vi "Do Action.vi"(8 "error in (no error)":errorcluster, 11 "Stand in":refnum<class "Stand.lvclass">) -> (0 "error out":errorcluster, 3 "Stand out":refnum<class "Stand.lvclass">)   [LabVIEW 2019, in "Stand.lvclass"]
uses:
  Stand.lvclass
  C:/Users/ANENKOV_V1/Desktop/src/Device_class/Device.lvclass
  Stand.lvclass/Stand.ctl
  TypeDef/Action.ctl
  FPGA/TypeDef/DO index.ctl
  Device_class/Device.lvclass/Device.ctl
  TypeDef/Active Motor.ctl
  TypeDef/Motor N.ctl
  AO_class/AO.lvclass/AO.ctl
  AI_class/AI.lvclass/AI.ctl
  AnalogComparator_class/AnalogComparator.lvclass/AnalogComparator.ctl
  OscillationClass/OscillationDetector.lvclass/OscillationDetector.ctl
  Valve_2DO_2DI_class/CMD.ctl
  NeedleValve_class/Cmd.ctl
  FPGA/TypeDef/AI index.ctl
  PM_Group_class/PM_Group.lvclass/PM_Group.ctl
  NeedleValve_class/NeedleValve.lvclass/NeedleValve.ctl
  TypeDef/Direction.ctl
  d1e0c5f4-8af3-4e63-9d82-d6085af126e6.vi
  AnalogComparator_class/GetStatus.vi
  FPGA_API_class/FPGA API.lvclass
  Device_class/Device.lvclass
  PM_Group_class/PM_Group.lvclass
  Valve_2DO_2DI_class/Valve_2DO_2DI.lvclass
  NeedleValve_class/NeedleValve.lvclass
  AI_class/AI.lvclass
  AO_class/AO.lvclass
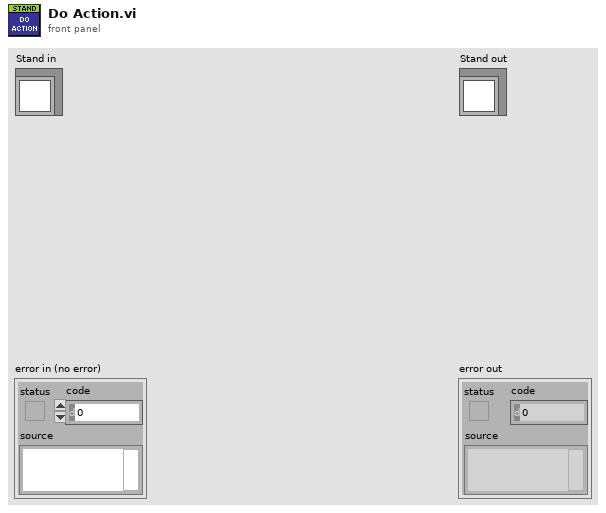
[diagram p1: front panel]
types:
  T1 = typedef "Action.ctl" = enum16{"Air: On", "Air: Off", "Pump Station: On (Filling Mode)", "Pump Station: On (Pressure Mode)", "Pump Station: Off", "Air Valves: Open (DUT Filling)", "Air Valves: Open (Chamber Filling)", "Air Valves: Open (Pump Pressure DUT)", "Air Valves: Open (Pump Pressure Chamber)", "Air Valves: Open (Haskel Pressure DUT)", "Air Valves: Open (Haskel Pressure Chamber)", "Air Valves: Open (Slow Release DUT)", "Air Valves: Open (Slow Release Chamber)", "Air Valves: Open (Fast Release DUT)", "Air Valves: Open (Fast Release Chamber)", "Air Valves: Open (Emergency Release DUT and Chamber)", "Air Valves: Open (Leak Test Pressure Sensor 41.3)", "Air Valves: Open (Leak Test Burette 42)", "Air Valves: Fully Closed", "Haskel: Off (0)", "Haskel: Pressure Control (PI Regulator)", "Haskel: Measure T0", "Proportional Valve: Off (0)", "Proportional Valve: Pressure Control (PI Regulator)", "Proportional Valve: Measure T0 DUT", "Valve 44.1: Open", "Valve 44.1: Close", "Valve 44.2: Open", "Valve 44.2: Close", "Valve 37.1: Open", "Valve 37.1: Close", "Valve 37.2: Open", "Valve 37.2: Close", "Filling: In Progress DUT", "Filling: In Progress Chamber", "Pressure pre loading: DUT", "Pressure pre loading: Chamber", "Slow Pressure Release: In Progress (DUT)", "Slow Pressure Release: In Progress (Chamber)", "NONE"}
  T2 = typedef "Active Motor.ctl" = cluster{"Active":bool, "MotorN":T3}
  T3 = typedef "Motor N.ctl" = enum16{"M12", "M21", "M24"}
  T4 = typedef "Valve_2DO_2DI.lvclass/CMD.ctl" = enum16{"Open", "Close"}
  T5 = typedef "NeedleValve.lvclass/Cmd.ctl" = enum16{"Open", "Close", "Stop"}
  T6 = typedef "Direction.ctl" = enum16{"None", "DUT", "Chamber"}
  T7 = typedef "DO index.ctl" = u8
  T8 = typedef "Setting Pressure PI.ctl" = cluster{"A [MPa/V]":dbl, "P start [MPa]":dbl, "P end [MPa]":dbl, "T0 DUT [s]":dbl, "T0 CMBR [s]":dbl}
  T9 = typedef "AI_Data.ctl" = cluster{"Stat Data":T10, "OutOfRangeMax":bool, "OutOfRangeMin":bool, "HIHI":bool, "HI":bool, "LO":bool, "LOLO":bool, "DATA N":T11, "DATA PERIOD":T11, "UPPER TH":dbl, "LOWER TH":dbl}
  T10 = typedef "AI Statistics Data.ctl" = cluster{"raw mean":dbl, "scl mean":dbl, "raw mean 1Hz":dbl, "scl mean 1Hz":dbl}
  T11 = typedef "DATA Oscill.ctl" = cluster{"SUM":dbl, "COUNTER":dbl, "MAX CURR":dbl, "MIN CURR":dbl, "AVR":dbl, "MAX":dbl, "MIN":dbl, "DELTA AVR":dbl, "DELTA MAX":dbl, "DELTA MIN":dbl, "PERIOD":dbl}
  T12 = typedef "AI index.ctl" = u8
  T13 = typedef "GUI Setting PMG.ctl" = cluster{"Temp Turn ON M24":dbl, "Temp Turn OFF M24":dbl, "Temp Open Water M21":dbl, "Temp Close Water M21":dbl, "delta level":dbl, "fililing level %":dbl, "fililing voltage [V]":dbl}
  T14 = typedef "Needle Valve Data.ctl" = cluster{"Engine State":T15, "StateValveModbus":T16, "Alarms":T17, "RAW":i32, "Angele":dbl, "Step":i32, "Encoder":i32, "Kinematic":T18, "Limits":T19, "EncoderMax":i32, "Counter Max Dont Update":i32, "EncoderMin":i32, "Counter Min Dont Update":i32, "Prepere Counter":i32, "STEP INIT":i32, "offset - Angel":dbl}
  T15 = typedef "MB_ENGINE.lvclass/Engine State.ctl" = u16
  T16 = typedef "Needle Valve State.ctl" = enum16{"STOPED", "CLOSED", "OPENED", "OPENING", "CLOSING"}
  T17 = typedef "MB_ENGINE.lvclass/Engine Alarms.ctl" = cluster{"OL":bool, "TF":bool, "STL":bool, "OCP":bool, "CPUV":bool, "UVLO":bool, "SPI_ERROR":bool, "Fault":bool, "OL 2":bool, "TF 2":bool, "STL 2":bool, "OCP 2":bool, "CPUV 2":bool, "UVLO 2":bool, "reserved":bool, "InitDone":bool}
  T18 = typedef "MB_ENGINE.lvclass/Settings.ctl" = cluster{"ACC Steps Per Sec^2":u16, "DEC Steps Per Sec^2":u16, "Min Velosity Step Per Sec":u16, "Max Velosity Step Per Sec":u16, "MicroStep":u16}
  T19 = typedef "MB_ENGINE.lvclass/Limits Status.ctl" = cluster{"Fault 2 Switch":bool, "Fault 1 Switch":bool, "Center(Home)":bool, "Lower Limit":bool, "Upper Limit":bool}
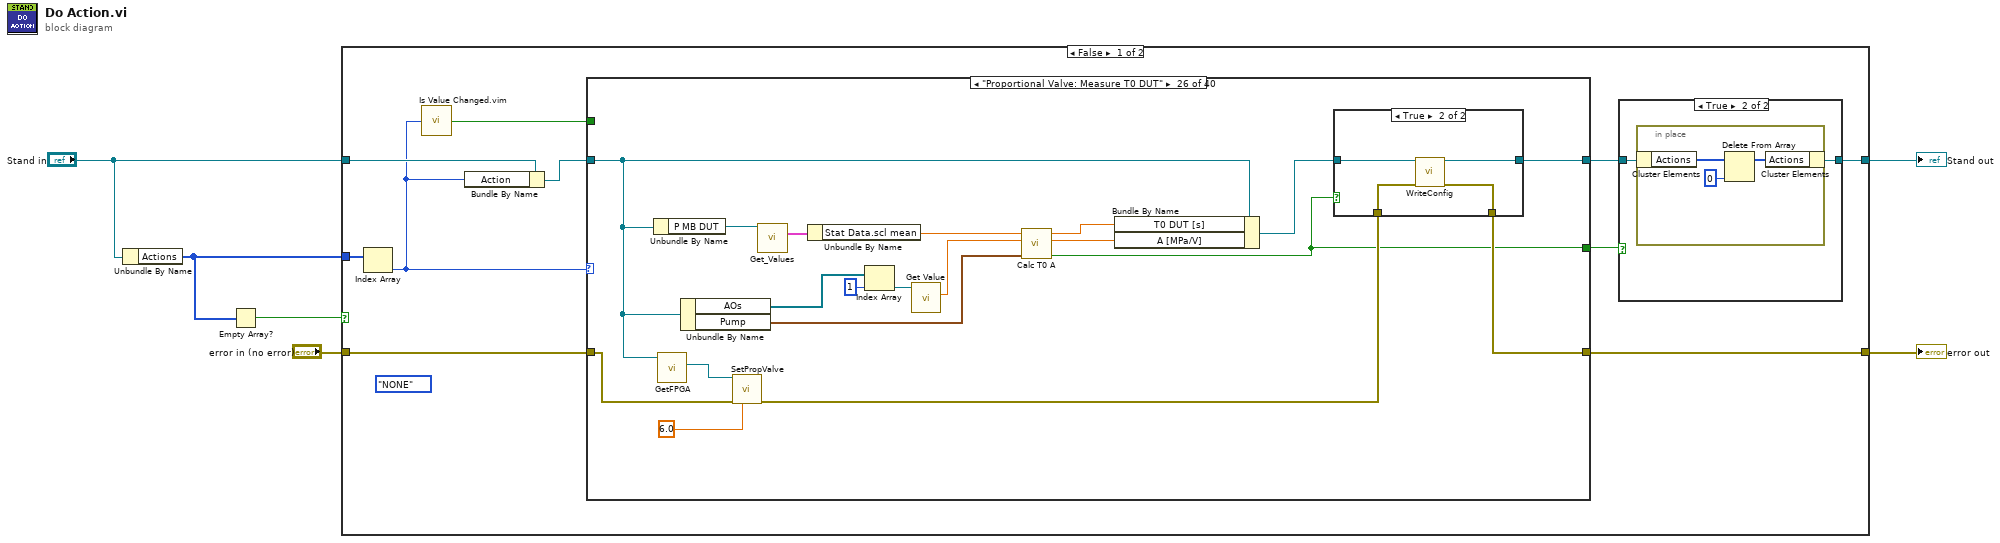
[diagram p0: block diagram]
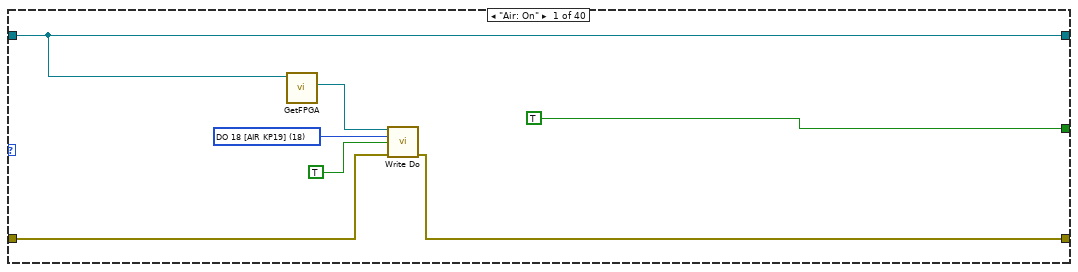
[diagram p2: hidden frame]
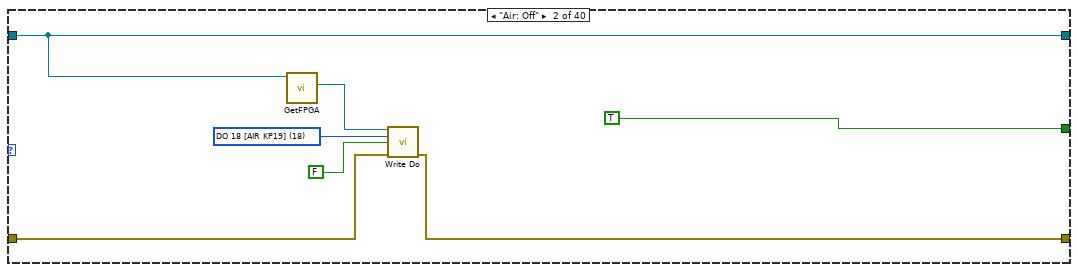
[diagram p3: hidden frame]
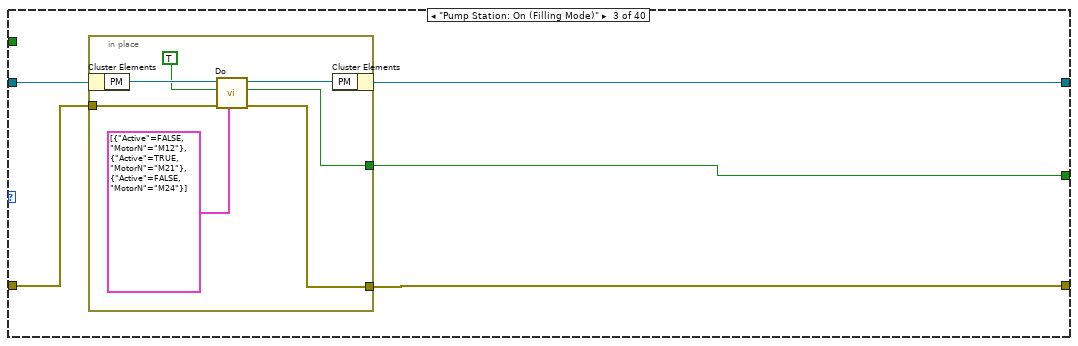
[diagram p4: hidden frame]
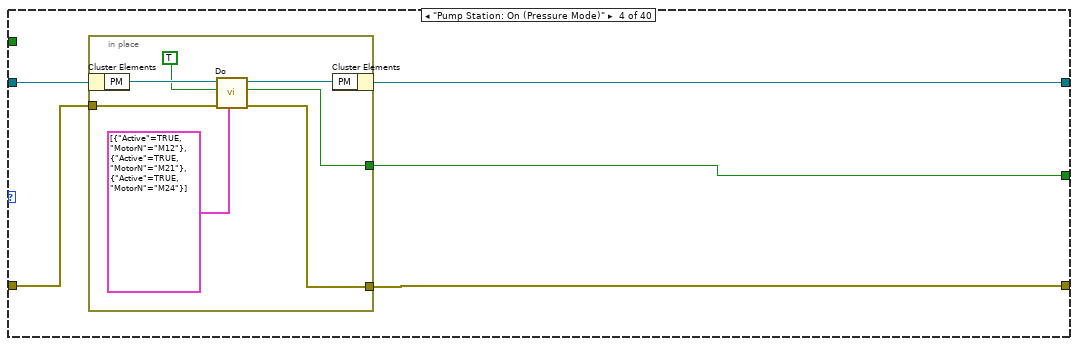
[diagram p5: hidden frame]
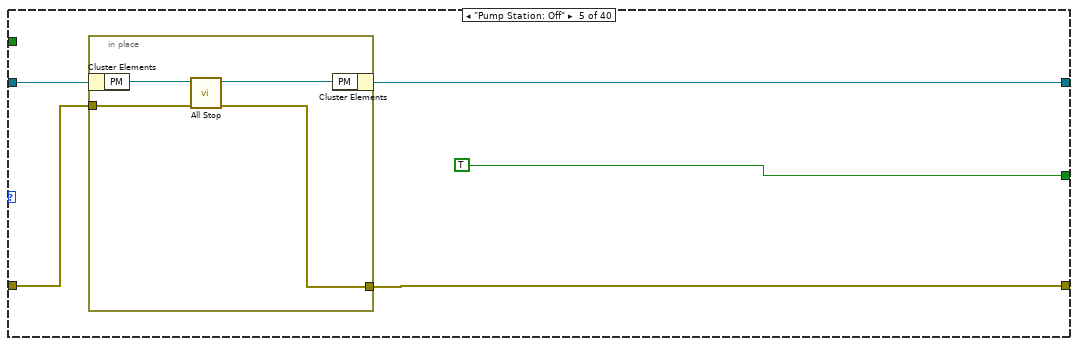
[diagram p6: hidden frame]
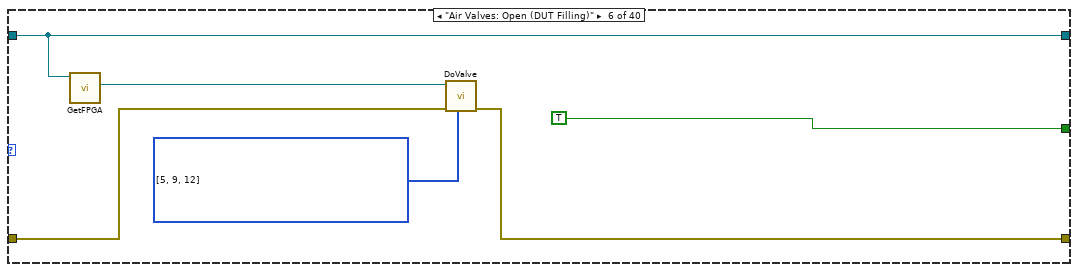
[diagram p7: hidden frame]
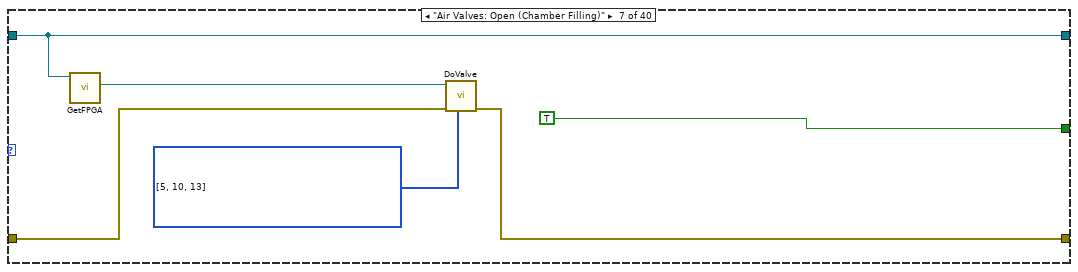
[diagram p8: hidden frame]
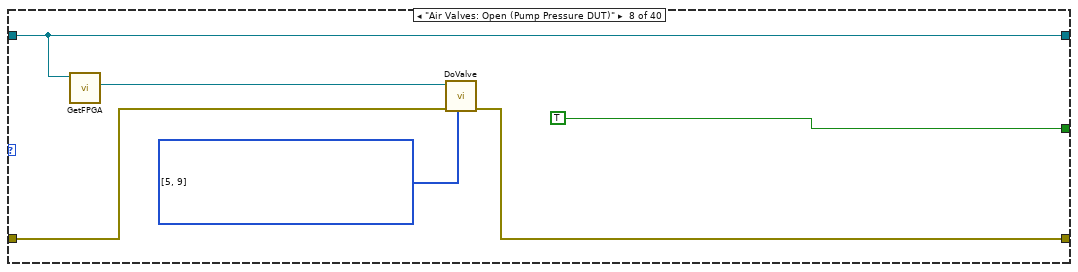
[diagram p9: hidden frame]
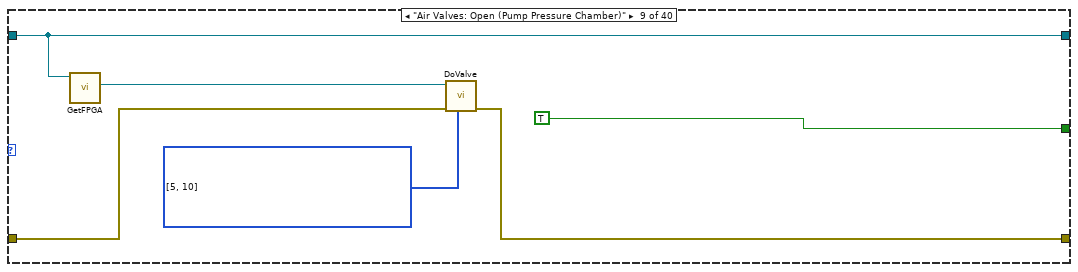
[diagram p10: hidden frame]
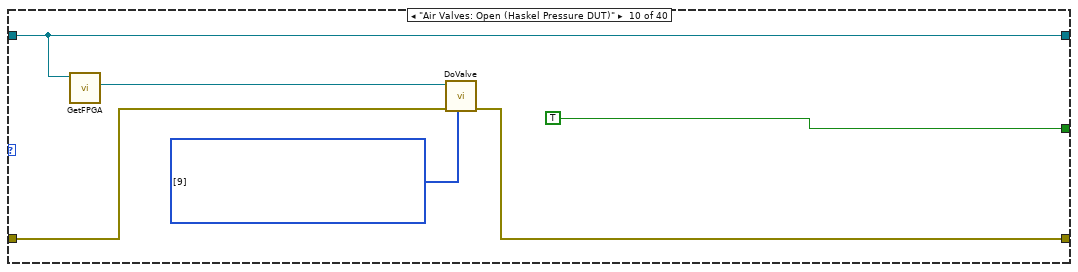
[diagram p11: hidden frame]
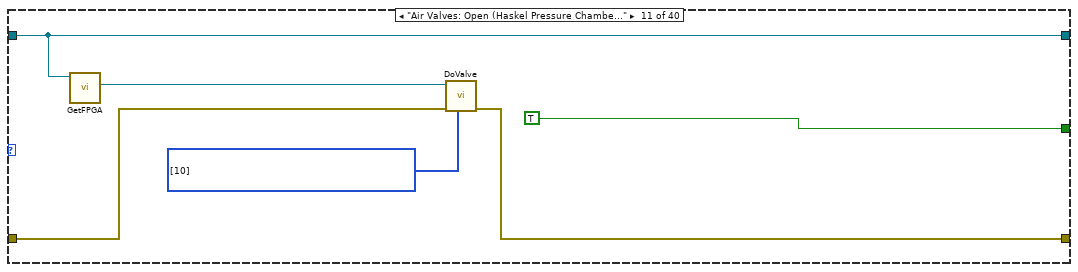
[diagram p12: hidden frame]
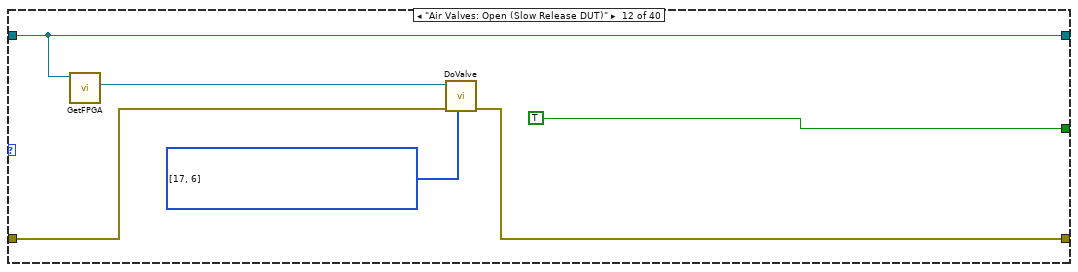
[diagram p13: hidden frame]
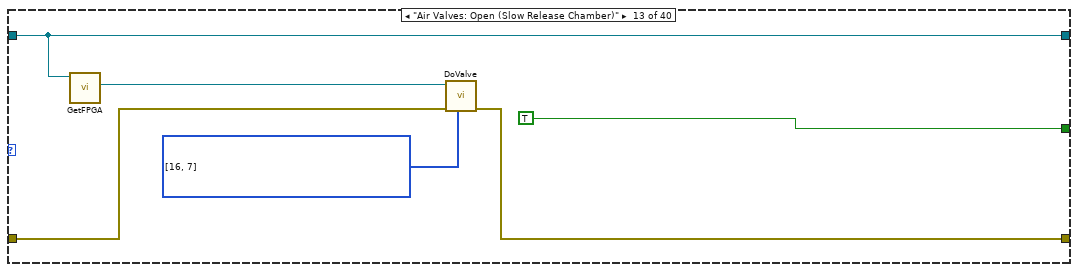
[diagram p14: hidden frame]
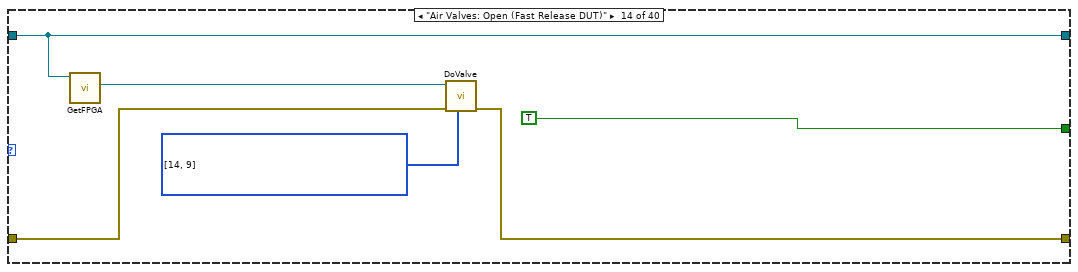
[diagram p15: hidden frame]
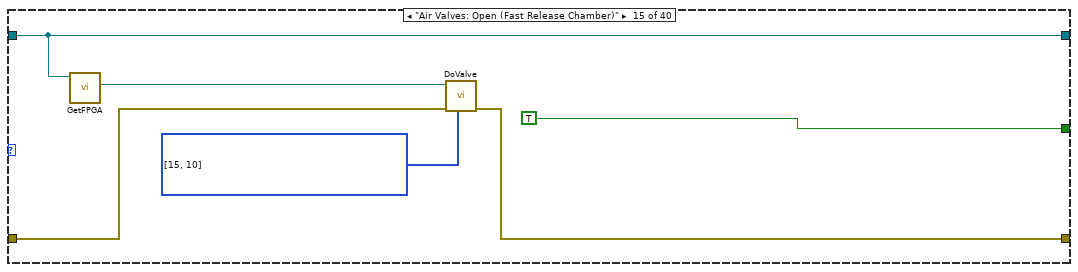
[diagram p16: hidden frame]
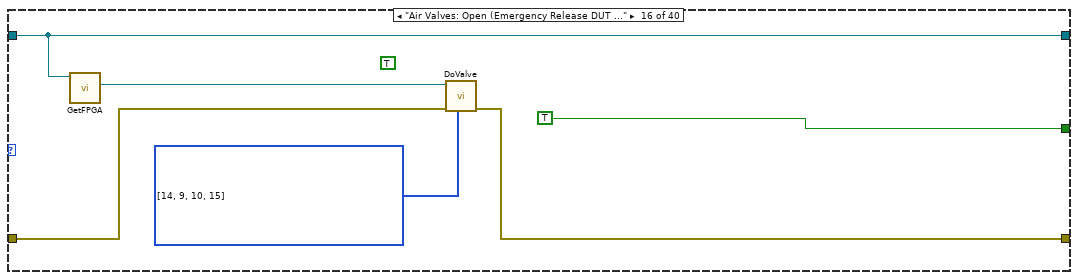
[diagram p17: hidden frame]
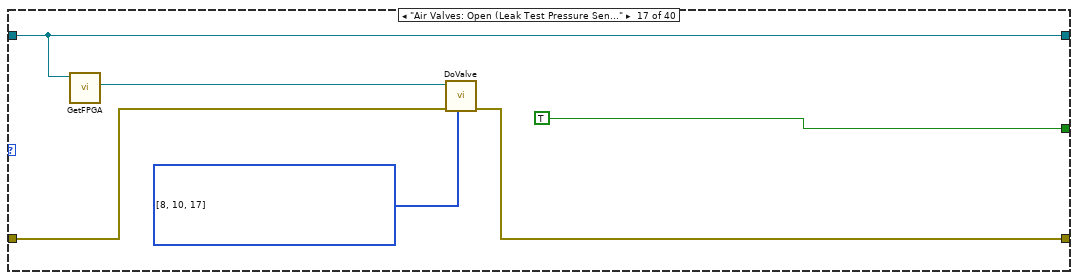
[diagram p18: hidden frame]
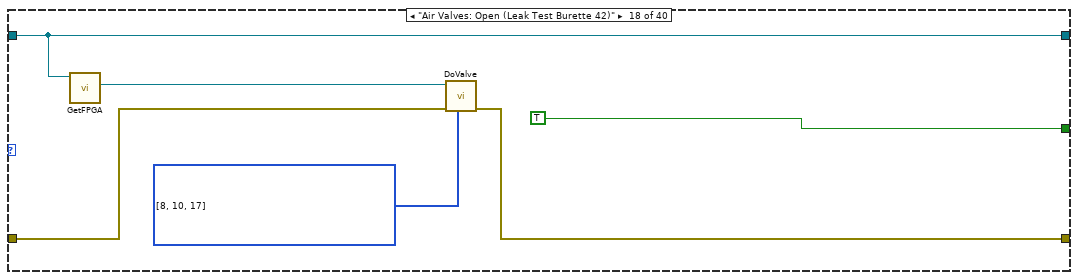
[diagram p19: hidden frame]
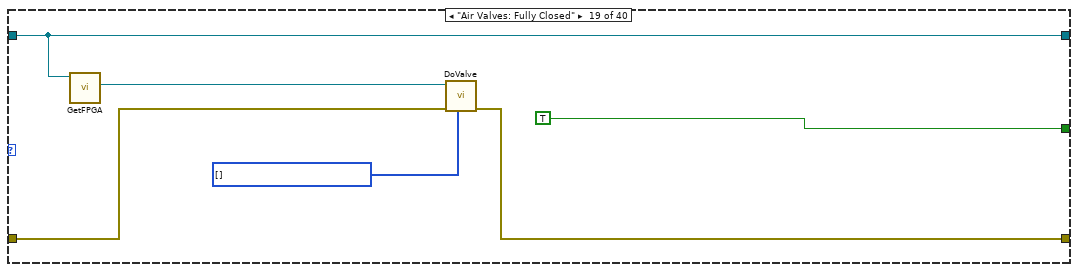
[diagram p20: hidden frame]
diagram:
  n1 = Unbundle By Name("Stand in") -> ("Actions"=w1:T1[])
  n2 = Empty Array?(array=w1) -> (empty?=w2:bool)
  n3 = case shown="False" w2 {
    tunnel: "Stand in" -> [w15 w477]
    tunnel: [w11 w475] -> w6
    tunnel: [w14 w476] -> w5
    tunnel: "error in (no error)" -> [w13 w476]
    tunnel: w1 -> [w16 _]
    frame False {
      (unwired) Action."NONE" ("Actions")
      n4 = Index Array(array=w16) -> (element=w7:T1)  [unwired: 1 in]
      n5 = call "Is Value Changed.vim"("value"=w7) -> ("changed or first call?"=w9:bool)
      n6 = Bundle By Name(cluster=w15, "Action"=w7) -> (w8:refnum<class "Stand.lvclass">)
      n7 = case shown="\"Proportional Valve: Measure T0 DUT\"" w7 {
        tunnel: [w23 w30 w32 w44 w56 w69 w75 w81 w87 w93 w99 w105 w111 w117 w123 w129 w135 w141 w147 w153 w156 w175 w179 w184 w189 w214 w233 w245 w257 w269 w283 w297 w311 w325 w337 w360 w385 w411 w434 w451] -> w10
        tunnel: w8 -> [w23 w30 w35 w47 w59 w69 w75 w81 w87 w93 w99 w105 w111 w117 w123 w129 w135 w141 w147 w153 w156 w175 w179 w184 w189 w218 w236 w248 w260 w272 w285 w299 w313 w327 w343 w366 w386 w412 w434 w451]
        tunnel: [w18 w25 w33 w45 w57 w64 w71 w77 w83 w89 w95 w101 w107 w113 w119 w125 w131 w137 w143 w148 w154 w174 w177 w181 w186 w213 w234 w246 w258 w270 w281 w295 w309 w323 w338 w361 w384 w410 w435 w452] -> w14
        tunnel: w13 -> [w19 w26 w34 w46 w58 w66 w72 w78 w84 w90 w96 w102 w108 w114 w120 w126 w132 w138 w144 w149 w157 w174 w177 w182 w187 w216 w235 w247 w259 w271 w284 w298 w312 w326 w339 w362 w383 w409 w436 w453]
        tunnel: [TRUE ("Done") TRUE ("Done") w31 w43 TRUE ("Done") TRUE ("Done") TRUE ("Done") TRUE ("Done") TRUE ("Done") TRUE ("Done") TRUE ("Done") TRUE ("Done") TRUE ("Done") TRUE ("Done") TRUE ("Done") TRUE ("Done") TRUE ("Done") TRUE ("Done") TRUE ("Done") TRUE ("Done") TRUE ("Done") TRUE ("Done") TRUE ("Done") TRUE ("Done") w190 w208 w232 w244 w256 w268 w280 w294 w308 w322 w336 w359 w382 w408 w443 w460] -> w12
        tunnel: w9 -> [_ _ _ _ _ _ _ _ _ _ _ _ _ _ _ _ _ _ _ _ w155 _ _ _ w188 _ _ _ _ _ w282 w296 w310 w324 w350 w373 _ _ _ _]
        frame "Air: On" {
          w22 = T7 18 items=["DO 0 [KP1] [M12]", "DO 1 [ON KP2] [M21]", "DO 2 [ON KP3] [M24]", "DO 3 [WATER Y18.1 [DO3]]", "DO 4 [WATER Y18.2 [DO4]]", "DO 5 [KP6 Y29.1 33.7]", "DO 6 [KP7 Y29.2 33.8]", "DO 7 [KP8 Y29.3 33.9]", "DO 8 [KP9 Y29.4  33.12]", "DO 9 [KP10 Y29.5 33.1]", "DO 10 [KP11 Y29.6 33.2]", "DO 11 [KP12 Y29.7  33.13]", "DO 12 [KP13 Y29.8  33.11]", "DO 13 [KP14 Y29.9 33.10]", "DO 14 [KP15 Y29.10  33.6]", "DO 15 [KP16 Y29.11  33.5]", "DO 16 [KP17 Y29.12  33.4]", "DO 17 [KP18 Y29.13 33.3]", "DO 18 [AIR KP19]", "DO 19 [STEP DRIVE EN KP20]", "DO 20 [KP21 Y44.1 OPEN]", "DO 21 [ KP22 Y44.1 CLOSE]", "DO 22 [ KP23 Y44.2 OPEN]", "DO 23", "DO 24 [STEP DRIVE 1]", "DO 25 [STEP DRIVE 2]"] ("#DO")
          n8 = call "GetFPGA.vi"("Device in"=w23) -> ("FPGA API.lvclass"=w21:refnum<class "FPGA API.lvclass">)  [unwired: 10 in]
          n9 = call-dynamic "Write Do.vi"("FPGA API in"=w21, "#DO"=w22, "value"=TRUE, "error in (no error)"=w19) -> ("error out"=w18:errorcluster)  [unwired: 10 in, 1 out]
        }
        frame "Air: Off" {
          w29 = T7 18 items=["DO 0 [KP1] [M12]", "DO 1 [ON KP2] [M21]", "DO 2 [ON KP3] [M24]", "DO 3 [WATER Y18.1 [DO3]]", "DO 4 [WATER Y18.2 [DO4]]", "DO 5 [KP6 Y29.1 33.7]", "DO 6 [KP7 Y29.2 33.8]", "DO 7 [KP8 Y29.3 33.9]", "DO 8 [KP9 Y29.4  33.12]", "DO 9 [KP10 Y29.5 33.1]", "DO 10 [KP11 Y29.6 33.2]", "DO 11 [KP12 Y29.7  33.13]", "DO 12 [KP13 Y29.8  33.11]", "DO 13 [KP14 Y29.9 33.10]", "DO 14 [KP15 Y29.10  33.6]", "DO 15 [KP16 Y29.11  33.5]", "DO 16 [KP17 Y29.12  33.4]", "DO 17 [KP18 Y29.13 33.3]", "DO 18 [AIR KP19]", "DO 19 [STEP DRIVE EN KP20]", "DO 20 [KP21 Y44.1 OPEN]", "DO 21 [ KP22 Y44.1 CLOSE]", "DO 22 [ KP23 Y44.2 OPEN]", "DO 23", "DO 24 [STEP DRIVE 1]", "DO 25 [STEP DRIVE 2]"] ("#DO")
          n10 = call "GetFPGA.vi"("Device in"=w30) -> ("FPGA API.lvclass"=w28:refnum<class "FPGA API.lvclass">)  [unwired: 10 in]
          n11 = call-dynamic "Write Do.vi"("FPGA API in"=w28, "#DO"=w29, "value"=FALSE, "error in (no error)"=w26) -> ("error out"=w25:errorcluster)  [unwired: 10 in, 1 out]
        }
        frame "Pump Station: On (Filling Mode)" {
          n12 = in-place {
            in-place-border: w34 -> [w41]
            in-place-border: [w39] -> w33
            in-place-border: [w36] -> w31
            n13 = in-place-cluster #1(w35) -> ("PM"=w42:refnum<class "PM_Group.lvclass">)
            n14 = call "Do.vi"("Data"=T2[] [{"Active"=FALSE, "MotorN"=enum."M12"}, {"Active"=TRUE, "MotorN"=enum."M21"}, {"Active"=FALSE, "MotorN"=enum."M24"}] ("Array"), "error in (no error)"=w41, "Do"=TRUE, "PM_Group in"=w42) -> ("error out"=w39:errorcluster, "Done"=w36:bool, "PM_Group out"=w40:refnum<class "PM_Group.lvclass">)  [unwired: 5 in]
            n15 = in-place-cluster #1("PM"=w40) -> (w32:refnum<class "Stand.lvclass">)
          }
        }
        frame "Pump Station: On (Pressure Mode)" {
          n16 = in-place {
            in-place-border: w46 -> [w53]
            in-place-border: [w51] -> w45
            in-place-border: [w48] -> w43
            n17 = in-place-cluster #2(w47) -> ("PM"=w54:refnum<class "PM_Group.lvclass">)
            n18 = call "Do.vi"("Data"=T2[] [{"Active"=TRUE, "MotorN"=enum."M12"}, {"Active"=TRUE, "MotorN"=enum."M21"}, {"Active"=TRUE, "MotorN"=enum."M24"}] ("Array"), "error in (no error)"=w53, "Do"=TRUE, "PM_Group in"=w54) -> ("error out"=w51:errorcluster, "Done"=w48:bool, "PM_Group out"=w52:refnum<class "PM_Group.lvclass">)  [unwired: 5 in]
            n19 = in-place-cluster #2("PM"=w52) -> (w44:refnum<class "Stand.lvclass">)
          }
        }
        frame "Pump Station: Off" {
          n20 = in-place {
            in-place-border: w58 -> [w62]
            in-place-border: [w60] -> w57
            n21 = in-place-cluster #3(w59) -> ("PM"=w63:refnum<class "PM_Group.lvclass">)
            n22 = call "All Stop.vi"("error in (no error)"=w62, "PM_Group in"=w63) -> ("error out"=w60:errorcluster, "PM_Group out"=w61:refnum<class "PM_Group.lvclass">)  [unwired: 8 in]
            n23 = in-place-cluster #3("PM"=w61) -> (w56:refnum<class "Stand.lvclass">)
          }
        }
        frame "Air Valves: Open (DUT Filling)" {
          w65 = T7[] [5, 9, 12] items=["DO 0 [KP1] [M12]", "DO 1 [ON KP2] [M21]", "DO 2 [ON KP3] [M24]", "DO 3 [WATER Y18.1 [DO3]]", "DO 4 [WATER Y18.2 [DO4]]", "DO 5 [KP6 Y29.1 33.7]", "DO 6 [KP7 Y29.2 33.8]", "DO 7 [KP8 Y29.3 33.9]", "DO 8 [KP9 Y29.4  33.12]", "DO 9 [KP10 Y29.5 33.1]", "DO 10 [KP11 Y29.6 33.2]", "DO 11 [KP12 Y29.7  33.13]", "DO 12 [KP13 Y29.8  33.11]", "DO 13 [KP14 Y29.9 33.10]", "DO 14 [KP15 Y29.10  33.6]", "DO 15 [KP16 Y29.11  33.5]", "DO 16 [KP17 Y29.12  33.4]", "DO 17 [KP18 Y29.13 33.3]", "DO 18 [AIR KP19]", "DO 19 [STEP DRIVE EN KP20]", "DO 20 [KP21 Y44.1 OPEN]", "DO 21 [ KP22 Y44.1 CLOSE]", "DO 22 [ KP23 Y44.2 OPEN]", "DO 23", "DO 24 [STEP DRIVE 1]", "DO 25 [STEP DRIVE 2]"] ("#DO")
          n24 = call "GetFPGA.vi"("Device in"=w69) -> ("FPGA API.lvclass"=w67:refnum<class "FPGA API.lvclass">)  [unwired: 10 in]
          n25 = call "DoValve.vi"("#DO"=w65, "error in (no error)"=w66, "reference in"=w67) -> ("error out"=w64:errorcluster)  [unwired: 7 in, 1 out]
        }
        frame "Air Valves: Open (Chamber Filling)" {
          w70 = T7[] [5, 10, 13] items=["DO 0 [KP1] [M12]", "DO 1 [ON KP2] [M21]", "DO 2 [ON KP3] [M24]", "DO 3 [WATER Y18.1 [DO3]]", "DO 4 [WATER Y18.2 [DO4]]", "DO 5 [KP6 Y29.1 33.7]", "DO 6 [KP7 Y29.2 33.8]", "DO 7 [KP8 Y29.3 33.9]", "DO 8 [KP9 Y29.4  33.12]", "DO 9 [KP10 Y29.5 33.1]", "DO 10 [KP11 Y29.6 33.2]", "DO 11 [KP12 Y29.7  33.13]", "DO 12 [KP13 Y29.8  33.11]", "DO 13 [KP14 Y29.9 33.10]", "DO 14 [KP15 Y29.10  33.6]", "DO 15 [KP16 Y29.11  33.5]", "DO 16 [KP17 Y29.12  33.4]", "DO 17 [KP18 Y29.13 33.3]", "DO 18 [AIR KP19]", "DO 19 [STEP DRIVE EN KP20]", "DO 20 [KP21 Y44.1 OPEN]", "DO 21 [ KP22 Y44.1 CLOSE]", "DO 22 [ KP23 Y44.2 OPEN]", "DO 23", "DO 24 [STEP DRIVE 1]", "DO 25 [STEP DRIVE 2]"] ("#DO")
          n26 = call "GetFPGA.vi"("Device in"=w75) -> ("FPGA API.lvclass"=w73:refnum<class "FPGA API.lvclass">)  [unwired: 10 in]
          n27 = call "DoValve.vi"("#DO"=w70, "error in (no error)"=w72, "reference in"=w73) -> ("error out"=w71:errorcluster)  [unwired: 7 in, 1 out]
        }
        frame "Air Valves: Open (Pump Pressure DUT)" {
          w76 = T7[] [5, 9] items=["DO 0 [KP1] [M12]", "DO 1 [ON KP2] [M21]", "DO 2 [ON KP3] [M24]", "DO 3 [WATER Y18.1 [DO3]]", "DO 4 [WATER Y18.2 [DO4]]", "DO 5 [KP6 Y29.1 33.7]", "DO 6 [KP7 Y29.2 33.8]", "DO 7 [KP8 Y29.3 33.9]", "DO 8 [KP9 Y29.4  33.12]", "DO 9 [KP10 Y29.5 33.1]", "DO 10 [KP11 Y29.6 33.2]", "DO 11 [KP12 Y29.7  33.13]", "DO 12 [KP13 Y29.8  33.11]", "DO 13 [KP14 Y29.9 33.10]", "DO 14 [KP15 Y29.10  33.6]", "DO 15 [KP16 Y29.11  33.5]", "DO 16 [KP17 Y29.12  33.4]", "DO 17 [KP18 Y29.13 33.3]", "DO 18 [AIR KP19]", "DO 19 [STEP DRIVE EN KP20]", "DO 20 [KP21 Y44.1 OPEN]", "DO 21 [ KP22 Y44.1 CLOSE]", "DO 22 [ KP23 Y44.2 OPEN]", "DO 23", "DO 24 [STEP DRIVE 1]", "DO 25 [STEP DRIVE 2]"] ("#DO")
          n28 = call "GetFPGA.vi"("Device in"=w81) -> ("FPGA API.lvclass"=w79:refnum<class "FPGA API.lvclass">)  [unwired: 10 in]
          n29 = call "DoValve.vi"("#DO"=w76, "error in (no error)"=w78, "reference in"=w79) -> ("error out"=w77:errorcluster)  [unwired: 7 in, 1 out]
        }
        frame "Air Valves: Open (Pump Pressure Chamber)" {
          w82 = T7[] [5, 10] items=["DO 0 [KP1] [M12]", "DO 1 [ON KP2] [M21]", "DO 2 [ON KP3] [M24]", "DO 3 [WATER Y18.1 [DO3]]", "DO 4 [WATER Y18.2 [DO4]]", "DO 5 [KP6 Y29.1 33.7]", "DO 6 [KP7 Y29.2 33.8]", "DO 7 [KP8 Y29.3 33.9]", "DO 8 [KP9 Y29.4  33.12]", "DO 9 [KP10 Y29.5 33.1]", "DO 10 [KP11 Y29.6 33.2]", "DO 11 [KP12 Y29.7  33.13]", "DO 12 [KP13 Y29.8  33.11]", "DO 13 [KP14 Y29.9 33.10]", "DO 14 [KP15 Y29.10  33.6]", "DO 15 [KP16 Y29.11  33.5]", "DO 16 [KP17 Y29.12  33.4]", "DO 17 [KP18 Y29.13 33.3]", "DO 18 [AIR KP19]", "DO 19 [STEP DRIVE EN KP20]", "DO 20 [KP21 Y44.1 OPEN]", "DO 21 [ KP22 Y44.1 CLOSE]", "DO 22 [ KP23 Y44.2 OPEN]", "DO 23", "DO 24 [STEP DRIVE 1]", "DO 25 [STEP DRIVE 2]"] ("#DO")
          n30 = call "GetFPGA.vi"("Device in"=w87) -> ("FPGA API.lvclass"=w85:refnum<class "FPGA API.lvclass">)  [unwired: 10 in]
          n31 = call "DoValve.vi"("#DO"=w82, "error in (no error)"=w84, "reference in"=w85) -> ("error out"=w83:errorcluster)  [unwired: 7 in, 1 out]
        }
        frame "Air Valves: Open (Haskel Pressure DUT)" {
          w88 = T7[] [9] items=["DO 0 [KP1] [M12]", "DO 1 [ON KP2] [M21]", "DO 2 [ON KP3] [M24]", "DO 3 [WATER Y18.1 [DO3]]", "DO 4 [WATER Y18.2 [DO4]]", "DO 5 [KP6 Y29.1 33.7]", "DO 6 [KP7 Y29.2 33.8]", "DO 7 [KP8 Y29.3 33.9]", "DO 8 [KP9 Y29.4  33.12]", "DO 9 [KP10 Y29.5 33.1]", "DO 10 [KP11 Y29.6 33.2]", "DO 11 [KP12 Y29.7  33.13]", "DO 12 [KP13 Y29.8  33.11]", "DO 13 [KP14 Y29.9 33.10]", "DO 14 [KP15 Y29.10  33.6]", "DO 15 [KP16 Y29.11  33.5]", "DO 16 [KP17 Y29.12  33.4]", "DO 17 [KP18 Y29.13 33.3]", "DO 18 [AIR KP19]", "DO 19 [STEP DRIVE EN KP20]", "DO 20 [KP21 Y44.1 OPEN]", "DO 21 [ KP22 Y44.1 CLOSE]", "DO 22 [ KP23 Y44.2 OPEN]", "DO 23", "DO 24 [STEP DRIVE 1]", "DO 25 [STEP DRIVE 2]"] ("#DO")
          n32 = call "GetFPGA.vi"("Device in"=w93) -> ("FPGA API.lvclass"=w91:refnum<class "FPGA API.lvclass">)  [unwired: 10 in]
          n33 = call "DoValve.vi"("#DO"=w88, "error in (no error)"=w90, "reference in"=w91) -> ("error out"=w89:errorcluster)  [unwired: 7 in, 1 out]
        }
        frame "Air Valves: Open (Haskel Pressure Chamber)" {
          w94 = T7[] [10] items=["DO 0 [KP1] [M12]", "DO 1 [ON KP2] [M21]", "DO 2 [ON KP3] [M24]", "DO 3 [WATER Y18.1 [DO3]]", "DO 4 [WATER Y18.2 [DO4]]", "DO 5 [KP6 Y29.1 33.7]", "DO 6 [KP7 Y29.2 33.8]", "DO 7 [KP8 Y29.3 33.9]", "DO 8 [KP9 Y29.4  33.12]", "DO 9 [KP10 Y29.5 33.1]", "DO 10 [KP11 Y29.6 33.2]", "DO 11 [KP12 Y29.7  33.13]", "DO 12 [KP13 Y29.8  33.11]", "DO 13 [KP14 Y29.9 33.10]", "DO 14 [KP15 Y29.10  33.6]", "DO 15 [KP16 Y29.11  33.5]", "DO 16 [KP17 Y29.12  33.4]", "DO 17 [KP18 Y29.13 33.3]", "DO 18 [AIR KP19]", "DO 19 [STEP DRIVE EN KP20]", "DO 20 [KP21 Y44.1 OPEN]", "DO 21 [ KP22 Y44.1 CLOSE]", "DO 22 [ KP23 Y44.2 OPEN]", "DO 23", "DO 24 [STEP DRIVE 1]", "DO 25 [STEP DRIVE 2]"] ("#DO")
          n34 = call "GetFPGA.vi"("Device in"=w99) -> ("FPGA API.lvclass"=w97:refnum<class "FPGA API.lvclass">)  [unwired: 10 in]
          n35 = call "DoValve.vi"("#DO"=w94, "error in (no error)"=w96, "reference in"=w97) -> ("error out"=w95:errorcluster)  [unwired: 7 in, 1 out]
        }
        frame "Air Valves: Open (Slow Release DUT)" {
          w100 = T7[] [17, 6] items=["DO 0 [KP1] [M12]", "DO 1 [ON KP2] [M21]", "DO 2 [ON KP3] [M24]", "DO 3 [WATER Y18.1 [DO3]]", "DO 4 [WATER Y18.2 [DO4]]", "DO 5 [KP6 Y29.1 33.7]", "DO 6 [KP7 Y29.2 33.8]", "DO 7 [KP8 Y29.3 33.9]", "DO 8 [KP9 Y29.4  33.12]", "DO 9 [KP10 Y29.5 33.1]", "DO 10 [KP11 Y29.6 33.2]", "DO 11 [KP12 Y29.7  33.13]", "DO 12 [KP13 Y29.8  33.11]", "DO 13 [KP14 Y29.9 33.10]", "DO 14 [KP15 Y29.10  33.6]", "DO 15 [KP16 Y29.11  33.5]", "DO 16 [KP17 Y29.12  33.4]", "DO 17 [KP18 Y29.13 33.3]", "DO 18 [AIR KP19]", "DO 19 [STEP DRIVE EN KP20]", "DO 20 [KP21 Y44.1 OPEN]", "DO 21 [ KP22 Y44.1 CLOSE]", "DO 22 [ KP23 Y44.2 OPEN]", "DO 23", "DO 24 [STEP DRIVE 1]", "DO 25 [STEP DRIVE 2]"] ("#DO")
          n36 = call "GetFPGA.vi"("Device in"=w105) -> ("FPGA API.lvclass"=w103:refnum<class "FPGA API.lvclass">)  [unwired: 10 in]
          n37 = call "DoValve.vi"("#DO"=w100, "error in (no error)"=w102, "reference in"=w103) -> ("error out"=w101:errorcluster)  [unwired: 7 in, 1 out]
        }
        frame "Air Valves: Open (Slow Release Chamber)" {
          w106 = T7[] [16, 7] items=["DO 0 [KP1] [M12]", "DO 1 [ON KP2] [M21]", "DO 2 [ON KP3] [M24]", "DO 3 [WATER Y18.1 [DO3]]", "DO 4 [WATER Y18.2 [DO4]]", "DO 5 [KP6 Y29.1 33.7]", "DO 6 [KP7 Y29.2 33.8]", "DO 7 [KP8 Y29.3 33.9]", "DO 8 [KP9 Y29.4  33.12]", "DO 9 [KP10 Y29.5 33.1]", "DO 10 [KP11 Y29.6 33.2]", "DO 11 [KP12 Y29.7  33.13]", "DO 12 [KP13 Y29.8  33.11]", "DO 13 [KP14 Y29.9 33.10]", "DO 14 [KP15 Y29.10  33.6]", "DO 15 [KP16 Y29.11  33.5]", "DO 16 [KP17 Y29.12  33.4]", "DO 17 [KP18 Y29.13 33.3]", "DO 18 [AIR KP19]", "DO 19 [STEP DRIVE EN KP20]", "DO 20 [KP21 Y44.1 OPEN]", "DO 21 [ KP22 Y44.1 CLOSE]", "DO 22 [ KP23 Y44.2 OPEN]", "DO 23", "DO 24 [STEP DRIVE 1]", "DO 25 [STEP DRIVE 2]"] ("#DO")
          n38 = call "GetFPGA.vi"("Device in"=w111) -> ("FPGA API.lvclass"=w109:refnum<class "FPGA API.lvclass">)  [unwired: 10 in]
          n39 = call "DoValve.vi"("#DO"=w106, "error in (no error)"=w108, "reference in"=w109) -> ("error out"=w107:errorcluster)  [unwired: 7 in, 1 out]
        }
        frame "Air Valves: Open (Fast Release DUT)" {
          w112 = T7[] [14, 9] items=["DO 0 [KP1] [M12]", "DO 1 [ON KP2] [M21]", "DO 2 [ON KP3] [M24]", "DO 3 [WATER Y18.1 [DO3]]", "DO 4 [WATER Y18.2 [DO4]]", "DO 5 [KP6 Y29.1 33.7]", "DO 6 [KP7 Y29.2 33.8]", "DO 7 [KP8 Y29.3 33.9]", "DO 8 [KP9 Y29.4  33.12]", "DO 9 [KP10 Y29.5 33.1]", "DO 10 [KP11 Y29.6 33.2]", "DO 11 [KP12 Y29.7  33.13]", "DO 12 [KP13 Y29.8  33.11]", "DO 13 [KP14 Y29.9 33.10]", "DO 14 [KP15 Y29.10  33.6]", "DO 15 [KP16 Y29.11  33.5]", "DO 16 [KP17 Y29.12  33.4]", "DO 17 [KP18 Y29.13 33.3]", "DO 18 [AIR KP19]", "DO 19 [STEP DRIVE EN KP20]", "DO 20 [KP21 Y44.1 OPEN]", "DO 21 [ KP22 Y44.1 CLOSE]", "DO 22 [ KP23 Y44.2 OPEN]", "DO 23", "DO 24 [STEP DRIVE 1]", "DO 25 [STEP DRIVE 2]"] ("#DO")
          n40 = call "GetFPGA.vi"("Device in"=w117) -> ("FPGA API.lvclass"=w115:refnum<class "FPGA API.lvclass">)  [unwired: 10 in]
          n41 = call "DoValve.vi"("#DO"=w112, "error in (no error)"=w114, "reference in"=w115) -> ("error out"=w113:errorcluster)  [unwired: 7 in, 1 out]
        }
        frame "Air Valves: Open (Fast Release Chamber)" {
          w118 = T7[] [15, 10] items=["DO 0 [KP1] [M12]", "DO 1 [ON KP2] [M21]", "DO 2 [ON KP3] [M24]", "DO 3 [WATER Y18.1 [DO3]]", "DO 4 [WATER Y18.2 [DO4]]", "DO 5 [KP6 Y29.1 33.7]", "DO 6 [KP7 Y29.2 33.8]", "DO 7 [KP8 Y29.3 33.9]", "DO 8 [KP9 Y29.4  33.12]", "DO 9 [KP10 Y29.5 33.1]", "DO 10 [KP11 Y29.6 33.2]", "DO 11 [KP12 Y29.7  33.13]", "DO 12 [KP13 Y29.8  33.11]", "DO 13 [KP14 Y29.9 33.10]", "DO 14 [KP15 Y29.10  33.6]", "DO 15 [KP16 Y29.11  33.5]", "DO 16 [KP17 Y29.12  33.4]", "DO 17 [KP18 Y29.13 33.3]", "DO 18 [AIR KP19]", "DO 19 [STEP DRIVE EN KP20]", "DO 20 [KP21 Y44.1 OPEN]", "DO 21 [ KP22 Y44.1 CLOSE]", "DO 22 [ KP23 Y44.2 OPEN]", "DO 23", "DO 24 [STEP DRIVE 1]", "DO 25 [STEP DRIVE 2]"] ("#DO")
          n42 = call "GetFPGA.vi"("Device in"=w123) -> ("FPGA API.lvclass"=w121:refnum<class "FPGA API.lvclass">)  [unwired: 10 in]
          n43 = call "DoValve.vi"("#DO"=w118, "error in (no error)"=w120, "reference in"=w121) -> ("error out"=w119:errorcluster)  [unwired: 7 in, 1 out]
        }
        frame "Air Valves: Open (Emergency Release DUT and Chamber)" {
          (unwired) TRUE ("Init")
          w124 = T7[] [14, 9, 10, 15] items=["DO 0 [KP1] [M12]", "DO 1 [ON KP2] [M21]", "DO 2 [ON KP3] [M24]", "DO 3 [WATER Y18.1 [DO3]]", "DO 4 [WATER Y18.2 [DO4]]", "DO 5 [KP6 Y29.1 33.7]", "DO 6 [KP7 Y29.2 33.8]", "DO 7 [KP8 Y29.3 33.9]", "DO 8 [KP9 Y29.4  33.12]", "DO 9 [KP10 Y29.5 33.1]", "DO 10 [KP11 Y29.6 33.2]", "DO 11 [KP12 Y29.7  33.13]", "DO 12 [KP13 Y29.8  33.11]", "DO 13 [KP14 Y29.9 33.10]", "DO 14 [KP15 Y29.10  33.6]", "DO 15 [KP16 Y29.11  33.5]", "DO 16 [KP17 Y29.12  33.4]", "DO 17 [KP18 Y29.13 33.3]", "DO 18 [AIR KP19]", "DO 19 [STEP DRIVE EN KP20]", "DO 20 [KP21 Y44.1 OPEN]", "DO 21 [ KP22 Y44.1 CLOSE]", "DO 22 [ KP23 Y44.2 OPEN]", "DO 23", "DO 24 [STEP DRIVE 1]", "DO 25 [STEP DRIVE 2]"] ("#DO")
          n44 = call "GetFPGA.vi"("Device in"=w129) -> ("FPGA API.lvclass"=w127:refnum<class "FPGA API.lvclass">)  [unwired: 10 in]
          n45 = call "DoValve.vi"("#DO"=w124, "error in (no error)"=w126, "reference in"=w127) -> ("error out"=w125:errorcluster)  [unwired: 7 in, 1 out]
        }
        frame "Air Valves: Open (Leak Test Pressure Sensor 41.3)" {
          w130 = T7[] [8, 10, 17] items=["DO 0 [KP1] [M12]", "DO 1 [ON KP2] [M21]", "DO 2 [ON KP3] [M24]", "DO 3 [WATER Y18.1 [DO3]]", "DO 4 [WATER Y18.2 [DO4]]", "DO 5 [KP6 Y29.1 33.7]", "DO 6 [KP7 Y29.2 33.8]", "DO 7 [KP8 Y29.3 33.9]", "DO 8 [KP9 Y29.4  33.12]", "DO 9 [KP10 Y29.5 33.1]", "DO 10 [KP11 Y29.6 33.2]", "DO 11 [KP12 Y29.7  33.13]", "DO 12 [KP13 Y29.8  33.11]", "DO 13 [KP14 Y29.9 33.10]", "DO 14 [KP15 Y29.10  33.6]", "DO 15 [KP16 Y29.11  33.5]", "DO 16 [KP17 Y29.12  33.4]", "DO 17 [KP18 Y29.13 33.3]", "DO 18 [AIR KP19]", "DO 19 [STEP DRIVE EN KP20]", "DO 20 [KP21 Y44.1 OPEN]", "DO 21 [ KP22 Y44.1 CLOSE]", "DO 22 [ KP23 Y44.2 OPEN]", "DO 23", "DO 24 [STEP DRIVE 1]", "DO 25 [STEP DRIVE 2]"] ("#DO")
          n46 = call "GetFPGA.vi"("Device in"=w135) -> ("FPGA API.lvclass"=w133:refnum<class "FPGA API.lvclass">)  [unwired: 10 in]
          n47 = call "DoValve.vi"("#DO"=w130, "error in (no error)"=w132, "reference in"=w133) -> ("error out"=w131:errorcluster)  [unwired: 7 in, 1 out]
        }
        frame "Air Valves: Open (Leak Test Burette 42)" {
          w136 = T7[] [8, 10, 17] items=["DO 0 [KP1] [M12]", "DO 1 [ON KP2] [M21]", "DO 2 [ON KP3] [M24]", "DO 3 [WATER Y18.1 [DO3]]", "DO 4 [WATER Y18.2 [DO4]]", "DO 5 [KP6 Y29.1 33.7]", "DO 6 [KP7 Y29.2 33.8]", "DO 7 [KP8 Y29.3 33.9]", "DO 8 [KP9 Y29.4  33.12]", "DO 9 [KP10 Y29.5 33.1]", "DO 10 [KP11 Y29.6 33.2]", "DO 11 [KP12 Y29.7  33.13]", "DO 12 [KP13 Y29.8  33.11]", "DO 13 [KP14 Y29.9 33.10]", "DO 14 [KP15 Y29.10  33.6]", "DO 15 [KP16 Y29.11  33.5]", "DO 16 [KP17 Y29.12  33.4]", "DO 17 [KP18 Y29.13 33.3]", "DO 18 [AIR KP19]", "DO 19 [STEP DRIVE EN KP20]", "DO 20 [KP21 Y44.1 OPEN]", "DO 21 [ KP22 Y44.1 CLOSE]", "DO 22 [ KP23 Y44.2 OPEN]", "DO 23", "DO 24 [STEP DRIVE 1]", "DO 25 [STEP DRIVE 2]"] ("#DO")
          n48 = call "GetFPGA.vi"("Device in"=w141) -> ("FPGA API.lvclass"=w139:refnum<class "FPGA API.lvclass">)  [unwired: 10 in]
          n49 = call "DoValve.vi"("#DO"=w136, "error in (no error)"=w138, "reference in"=w139) -> ("error out"=w137:errorcluster)  [unwired: 7 in, 1 out]
        }
        frame "Air Valves: Fully Closed" {
          w142 = T7[] [] items=["DO 0 [KP1] [M12]", "DO 1 [ON KP2] [M21]", "DO 2 [ON KP3] [M24]", "DO 3 [WATER Y18.1 [DO3]]", "DO 4 [WATER Y18.2 [DO4]]", "DO 5 [KP6 Y29.1 33.7]", "DO 6 [KP7 Y29.2 33.8]", "DO 7 [KP8 Y29.3 33.9]", "DO 8 [KP9 Y29.4  33.12]", "DO 9 [KP10 Y29.5 33.1]", "DO 10 [KP11 Y29.6 33.2]", "DO 11 [KP12 Y29.7  33.13]", "DO 12 [KP13 Y29.8  33.11]", "DO 13 [KP14 Y29.9 33.10]", "DO 14 [KP15 Y29.10  33.6]", "DO 15 [KP16 Y29.11  33.5]", "DO 16 [KP17 Y29.12  33.4]", "DO 17 [KP18 Y29.13 33.3]", "DO 18 [AIR KP19]", "DO 19 [STEP DRIVE EN KP20]", "DO 20 [KP21 Y44.1 OPEN]", "DO 21 [ KP22 Y44.1 CLOSE]", "DO 22 [ KP23 Y44.2 OPEN]", "DO 23", "DO 24 [STEP DRIVE 1]", "DO 25 [STEP DRIVE 2]"] ("#DO")
          n50 = call "GetFPGA.vi"("Device in"=w147) -> ("FPGA API.lvclass"=w145:refnum<class "FPGA API.lvclass">)  [unwired: 10 in]
          n51 = call "DoValve.vi"("#DO"=w142, "error in (no error)"=w144, "reference in"=w145) -> ("error out"=w143:errorcluster)  [unwired: 7 in, 1 out]
        }
        frame "Haskel: Off (0)" {
          n52 = call "GetFPGA.vi"("Device in"=w153) -> ("FPGA API.lvclass"=w151:refnum<class "FPGA API.lvclass">)  [unwired: 10 in]
          n53 = call-dynamic "SetHasckelAO.vi"("FPGA API in"=w151, "Haskel in"=0.0, "error in (no error)"=w149) -> ("error out"=w148:errorcluster)  [unwired: 11 in, 1 out]
        }
        frame "Haskel: Pressure Control (PI Regulator)" {
          n54 = disable-structure shown="Disabled" {
            disable-tunnel: w157 -> [w162 _]
            disable-tunnel: w156 -> [w161 _]
            disable-tunnel: w155 -> [w160 _]
            disable-tunnel: [w159 _] -> w154
            frame Disabled {
              n55 = call "GetFPGA.vi"("Device in"=w161) -> ("FPGA API.lvclass"=w163:refnum<class "FPGA API.lvclass">)  [unwired: 10 in]
              n56 = Unbundle By Name(w161) -> ("Pressure SP"=w173:dbl)
              n57 = call "Get PV.vi"("Stand in"=w161) -> ("Stat Data.scl mean"=w172:dbl)  [unwired: 10 in]
              n58 = Unbundle By Name(w161) -> ("A Haskel [MPa/V]"=w171:dbl, "T0 Haslel DUT"=w165:dbl)
              n59 = call "Loop Time Const.vi"() -> ("loop time ms"=w168:i64)  [unwired: 3 in]
              n60 = Divide(x=w168, y=i64 1000) -> (x/y=w166:dbl)
              n61 = call "PI_Controller.vi"("SP"=w173, "Init"=w160, "PV"=w172, "A"=w171, "T0"=w165, "dt"=w166, "U min"=0.0, "U max"=5.0) -> ("U out"=w164:dbl)  [unwired: 7 in]
              n62 = call-dynamic "SetHasckelAO.vi"("FPGA API in"=w163, "Haskel in"=w164, "error in (no error)"=w162) -> ("error out"=w159:errorcluster)  [unwired: 11 in, 1 out]
            }
            frame Enabled {
            }
          }
        }
        frame "Haskel: Measure T0" {
          n63 = call "GetFPGA.vi"("Device in"=w175) -> ()  [unwired: 10 in, 1 out]
        }
        frame "NONE" {
        }
        frame "Proportional Valve: Off (0)" {
          n64 = call "GetFPGA.vi"("Device in"=w184) -> ("FPGA API.lvclass"=w183:refnum<class "FPGA API.lvclass">)  [unwired: 10 in]
          n65 = call-dynamic "SetPropValve.vi"("FPGA API in"=w183, "error in (no error)"=w182, "AO 1"=0.0) -> ("error out"=w181:errorcluster)  [unwired: 11 in, 1 out]
        }
        frame "Proportional Valve: Pressure Control (PI Regulator)" {
          n66 = disable-structure shown="Disabled" {
            disable-tunnel: [TRUE ("Done") _] -> w190
            disable-tunnel: w189 -> [w196 _]
            disable-tunnel: w188 -> [w195 _]
            disable-tunnel: w187 -> [w194 _]
            disable-tunnel: [w191 _] -> w186
            frame Disabled {
              (unwired) TRUE ("Init")
              # "#Get T0"
              n67 = call "GetFPGA.vi"("Device in"=w196) -> ("FPGA API.lvclass"=w193:refnum<class "FPGA API.lvclass">)  [unwired: 10 in]
              n68 = Unbundle By Name(w196) -> ("Pressure SP"=w205:dbl)
              n69 = call "Get PV.vi"("Stand in"=w196) -> ("Stat Data.scl mean"=w204:dbl)  [unwired: 10 in]
              n70 = Unbundle By Name(w196) -> ("A Pump [MPa/V]"=w203:dbl, "T0 Haslel DUT"=w197:dbl)
              n71 = call "Loop Time Const.vi"() -> ("loop time ms"=w200:i64)  [unwired: 3 in]
              n72 = Divide(x=w200, y=i64 1000) -> (x/y=w198:dbl)
              n73 = call "PI_Controller.vi"("SP"=w205, "Init"=w195, "PV"=w204, "A"=w203, "T0"=w197, "dt"=w198, "U min"=0.0, "U max"=5.0) -> ("U out"=w192:dbl)  [unwired: 7 in]
              n74 = call-dynamic "SetPropValve.vi"("FPGA API in"=w193, "error in (no error)"=w194, "AO 1"=w192) -> ("error out"=w191:errorcluster)  [unwired: 11 in, 1 out]
            }
            frame Enabled {
            }
          }
        }
        frame "Proportional Valve: Measure T0 DUT" {
          n75 = Unbundle By Name(w218) -> ("P MB DUT"=w223:refnum<class "AI.lvclass">)
          n76 = call "GetFPGA.vi"("Device in"=w218) -> ("FPGA API.lvclass"=w224:refnum<class "FPGA API.lvclass">)  [unwired: 10 in]
          n77 = Unbundle By Name(w218) -> ("AOs"=w219:refnum<class "AO.lvclass">[], "Pump"=w211:T8)
          n78 = call-dynamic "SetPropValve.vi"("FPGA API in"=w224, "error in (no error)"=w216, "AO 1"=6.0) -> ("error out"=w212:errorcluster)  [unwired: 11 in, 1 out]
          n79 = call "Get_Values.vi"("reference in"=w223) -> ("Data"=w222:T9)  [unwired: 14 in]
          n80 = Unbundle By Name(w222) -> ("Stat Data.scl mean"=w210:dbl)
          n81 = Index Array(array=w219, index=1) -> (element=w220:refnum<class "AO.lvclass">)
          n82 = call "Get Value.vi"("AO in"=w220) -> ("Value"=w209:dbl)  [unwired: 10 in]
          n83 = call "Calc T0 A.vi"("Pump"=w211, "U"=w209, "P"=w210) -> ("done"=w208:bool, "A"=w207:dbl, "T0"=w217:dbl)  [unwired: 6 in]
          n84 = Bundle By Name(cluster=w218, "T0 DUT [s]"=w217, "A [MPa/V]"=w207) -> (w215:refnum<class "Stand.lvclass">)
          n85 = case shown="True" w208 {
            tunnel: w215 -> [w227 w231]
            tunnel: [w227 w230] -> w214
            tunnel: [w226 w229] -> w213
            tunnel: w212 -> [w226 w228]
            frame False {
            }
            frame True {
              n86 = call-dynamic "WriteConfig.vi"("reference in"=w231, "error in (no error)"=w228) -> ("reference out"=w230:refnum<class "Stand.lvclass">, "error out"=w229:errorcluster)  [unwired: 12 in]
            }
          }
        }
        frame "Valve 44.1: Open" {
          n87 = in-place {
            in-place-border: w235 -> [w241]
            in-place-border: [w239] -> w234
            in-place-border: [w237] -> w232
            n88 = in-place-cluster #4(w236) -> ("VLV 44.1"=w243:refnum<class "Valve_2DO_2DI.lvclass">)
            n89 = call "Do.vi"("CMD"=CMD."Open", "error in (no error)"=w241, "Do"=TRUE, "Valve_2DO_2DI in"=w243) -> ("error out"=w239:errorcluster, "Done"=w237:bool, "Valve_2DO_2DI out"=w242:refnum<class "Valve_2DO_2DI.lvclass">)  [unwired: 5 in]
            n90 = in-place-cluster #4("VLV 44.1"=w242) -> (w233:refnum<class "Stand.lvclass">)
          }
        }
        frame "Valve 44.1: Close" {
          n91 = in-place {
            in-place-border: w247 -> [w253]
            in-place-border: [w251] -> w246
            in-place-border: [w249] -> w244
            n92 = in-place-cluster #5(w248) -> ("VLV 44.1"=w255:refnum<class "Valve_2DO_2DI.lvclass">)
            n93 = call "Do.vi"("CMD"=CMD."Close", "error in (no error)"=w253, "Do"=TRUE, "Valve_2DO_2DI in"=w255) -> ("error out"=w251:errorcluster, "Done"=w249:bool, "Valve_2DO_2DI out"=w254:refnum<class "Valve_2DO_2DI.lvclass">)  [unwired: 5 in]
            n94 = in-place-cluster #5("VLV 44.1"=w254) -> (w245:refnum<class "Stand.lvclass">)
          }
        }
        frame "Valve 44.2: Open" {
          n95 = in-place {
            in-place-border: w259 -> [w265]
            in-place-border: [w263] -> w258
            in-place-border: [w261] -> w256
            n96 = in-place-cluster #6(w260) -> ("VLV 44.2"=w267:refnum<class "Valve_2DO_2DI.lvclass">)
            n97 = call "Do.vi"("CMD"=CMD."Open", "error in (no error)"=w265, "Do"=TRUE, "Valve_2DO_2DI in"=w267) -> ("error out"=w263:errorcluster, "Done"=w261:bool, "Valve_2DO_2DI out"=w266:refnum<class "Valve_2DO_2DI.lvclass">)  [unwired: 5 in]
            n98 = in-place-cluster #6("VLV 44.2"=w266) -> (w257:refnum<class "Stand.lvclass">)
          }
        }
        frame "Valve 44.2: Close" {
          n99 = in-place {
            in-place-border: w271 -> [w277]
            in-place-border: [w275] -> w270
            in-place-border: [w273] -> w268
            n100 = in-place-cluster #7(w272) -> ("VLV 44.2"=w279:refnum<class "Valve_2DO_2DI.lvclass">)
            n101 = call "Do.vi"("CMD"=CMD."Close", "error in (no error)"=w277, "Do"=TRUE, "Valve_2DO_2DI in"=w279) -> ("error out"=w275:errorcluster, "Done"=w273:bool, "Valve_2DO_2DI out"=w278:refnum<class "Valve_2DO_2DI.lvclass">)  [unwired: 5 in]
            n102 = in-place-cluster #7("VLV 44.2"=w278) -> (w269:refnum<class "Stand.lvclass">)
          }
        }
        frame "Valve 37.1: Open" {
          n103 = in-place {
            in-place-border: w284 -> [w289]
            in-place-border: w282 -> [w291]
            in-place-border: [w288] -> w281
            in-place-border: [w286] -> w280
            n104 = in-place-cluster #8(w285) -> ("NV_DUT"=w293:refnum<class "NeedleValve.lvclass">)
            n105 = call "Do.vi"("Cmd"=Cmd."Open", "init"=w291, "error in (no error)"=w289, "Do"=TRUE, "NeedleValve in"=w293) -> ("error out"=w288:errorcluster, "Done"=w286:bool, "NeedleValve out"=w292:refnum<class "NeedleValve.lvclass">)  [unwired: 4 in]
            n106 = in-place-cluster #8("NV_DUT"=w292) -> (w283:refnum<class "Stand.lvclass">)
          }
        }
        frame "Valve 37.1: Close" {
          n107 = in-place {
            in-place-border: w298 -> [w303]
            in-place-border: w296 -> [w305]
            in-place-border: [w302] -> w295
            in-place-border: [w300] -> w294
            n108 = in-place-cluster #9(w299) -> ("NV_DUT"=w307:refnum<class "NeedleValve.lvclass">)
            n109 = call "Do.vi"("Cmd"=Cmd."Close", "init"=w305, "error in (no error)"=w303, "Do"=TRUE, "NeedleValve in"=w307) -> ("error out"=w302:errorcluster, "Done"=w300:bool, "NeedleValve out"=w306:refnum<class "NeedleValve.lvclass">)  [unwired: 4 in]
            n110 = in-place-cluster #9("NV_DUT"=w306) -> (w297:refnum<class "Stand.lvclass">)
          }
        }
        frame "Valve 37.2: Open" {
          n111 = in-place {
            in-place-border: w312 -> [w317]
            in-place-border: w310 -> [w319]
            in-place-border: [w316] -> w309
            in-place-border: [w314] -> w308
            n112 = in-place-cluster #10(w313) -> ("NV_Chamber"=w321:refnum<class "NeedleValve.lvclass">)
            n113 = call "Do.vi"("Cmd"=Cmd."Open", "init"=w319, "error in (no error)"=w317, "Do"=TRUE, "NeedleValve in"=w321) -> ("error out"=w316:errorcluster, "Done"=w314:bool, "NeedleValve out"=w320:refnum<class "NeedleValve.lvclass">)  [unwired: 4 in]
            n114 = in-place-cluster #10("NV_Chamber"=w320) -> (w311:refnum<class "Stand.lvclass">)
          }
        }
        frame "Valve 37.2: Close" {
          n115 = in-place {
            in-place-border: w326 -> [w331]
            in-place-border: w324 -> [w333]
            in-place-border: [w330] -> w323
            in-place-border: [w328] -> w322
            n116 = in-place-cluster #11(w327) -> ("NV_Chamber"=w335:refnum<class "NeedleValve.lvclass">)
            n117 = call "Do.vi"("Cmd"=Cmd."Close", "init"=w333, "error in (no error)"=w331, "Do"=TRUE, "NeedleValve in"=w335) -> ("error out"=w330:errorcluster, "Done"=w328:bool, "NeedleValve out"=w334:refnum<class "NeedleValve.lvclass">)  [unwired: 4 in]
            n118 = in-place-cluster #11("NV_Chamber"=w334) -> (w325:refnum<class "Stand.lvclass">)
          }
        }
        frame "Filling: In Progress DUT" {
          w353 = T12 0 items=["AI 0 Cooling Station Level", "AI 1 Cooling Station Temp", "AI 2 Oil Supply Level", "AI 3 Oil Supply Temp", "AI 4 ", "AI 5 Pressure Haskel", "AI 6 Pressure DUT", "AI 7 Pressure Chamber", "AI 8 Pressure Air inlet", "AI 9 Pressure Air outlet", "AI 10 Pressure Messure Line"] ("AI index")
          n119 = Unbundle By Name(w343) -> ("PM"=w347:refnum<class "PM_Group.lvclass">)
          n120 = Unbundle By Name(w343) -> ("AIs"=w352:refnum<class "AI.lvclass">[])
          n121 = call "GetFPGA.vi"("Device in"=w343) -> ("FPGA API.lvclass"=w348:refnum<class "FPGA API.lvclass">)  [unwired: 10 in]
          n122 = call "Get Setting.vi"("PM_Group in"=w347) -> ("Setting PMG"=w345:T13)  [unwired: 9 in, 1 out]
          n123 = Index Array(array=w352, index=w353) -> (element=w351:refnum<class "AI.lvclass">)
          n124 = call "Get_Values.vi"("reference in"=w351) -> ("Data"=w354:T9)  [unwired: 14 in]
          n125 = Unbundle By Name(w345) -> ("fililing voltage [V]"=w344:dbl)
          n126 = Unbundle By Name(w354) -> ("Stat Data.scl mean 1Hz"=w340:dbl)
          n127 = call-dynamic "SetPropValve.vi"("FPGA API in"=w348, "error in (no error)"=w339, "AO 1"=w344) -> ("error out"=w338:errorcluster)  [unwired: 11 in, 1 out]
          n128 = case shown="True" w350 {
            tunnel: w340 -> [_ w358]
            tunnel: w343 -> [w355 w357]
            tunnel: [w355 w356] -> w349
            frame False {
            }
            frame True {
              n129 = Bundle By Name(cluster=w357, "BeginFilingLevel"=w358) -> (w356:refnum<class "Stand.lvclass">)
            }
          }
          n130 = Unbundle By Name(w349) -> ("BeginFilingLevel"=w342:dbl)
          n131 = Unbundle By Name(w345) -> ("fililing level %"=w346:dbl)
          n132 = Add(x=w342, y=w346) -> (x+y=w341:dbl)
          n133 = Greater?(x=w340, y=w341) -> (0:w336:bool)
          n134 = Bundle By Name(cluster=w349, "Filling Done DUT"=w336) -> (w337:refnum<class "Stand.lvclass">)
        }
        frame "Filling: In Progress Chamber" {
          w376 = T12 0 items=["AI 0 Cooling Station Level", "AI 1 Cooling Station Temp", "AI 2 Oil Supply Level", "AI 3 Oil Supply Temp", "AI 4 ", "AI 5 Pressure Haskel", "AI 6 Pressure DUT", "AI 7 Pressure Chamber", "AI 8 Pressure Air inlet", "AI 9 Pressure Air outlet", "AI 10 Pressure Messure Line"] ("AI index")
          n135 = Unbundle By Name(w366) -> ("PM"=w370:refnum<class "PM_Group.lvclass">)
          n136 = Unbundle By Name(w366) -> ("AIs"=w375:refnum<class "AI.lvclass">[])
          n137 = call "GetFPGA.vi"("Device in"=w366) -> ("FPGA API.lvclass"=w371:refnum<class "FPGA API.lvclass">)  [unwired: 10 in]
          n138 = call "Get Setting.vi"("PM_Group in"=w370) -> ("Setting PMG"=w368:T13)  [unwired: 9 in, 1 out]
          n139 = Index Array(array=w375, index=w376) -> (element=w374:refnum<class "AI.lvclass">)
          n140 = call "Get_Values.vi"("reference in"=w374) -> ("Data"=w377:T9)  [unwired: 14 in]
          n141 = Unbundle By Name(w368) -> ("fililing voltage [V]"=w367:dbl)
          n142 = Unbundle By Name(w377) -> ("Stat Data.scl mean 1Hz"=w363:dbl)
          n143 = call-dynamic "SetPropValve.vi"("FPGA API in"=w371, "error in (no error)"=w362, "AO 1"=w367) -> ("error out"=w361:errorcluster)  [unwired: 11 in, 1 out]
          n144 = case shown="True" w373 {
            tunnel: w363 -> [_ w381]
            tunnel: w366 -> [w378 w380]
            tunnel: [w378 w379] -> w372
            frame False {
            }
            frame True {
              n145 = Bundle By Name(cluster=w380, "BeginFilingLevel"=w381) -> (w379:refnum<class "Stand.lvclass">)
            }
          }
          n146 = Unbundle By Name(w372) -> ("BeginFilingLevel"=w365:dbl)
          n147 = Unbundle By Name(w368) -> ("fililing level %"=w369:dbl)
          n148 = Add(x=w365, y=w369) -> (x+y=w364:dbl)
          n149 = Greater?(x=w363, y=w364) -> (0:w359:bool)
          n150 = Bundle By Name(cluster=w372, "Filling Done CHMBR"=w359) -> (w360:refnum<class "Stand.lvclass">)
        }
        frame "Pressure pre loading: DUT" {
          n151 = call "Get PV.vi"("Stand in"=w386) -> ("Stat Data.scl mean"=w388:dbl)  [unwired: 10 in]
          n152 = Greater?(x=w388, y=3.0) -> (0:w382:bool)
          n153 = case shown="True" w382 {
            tunnel: w386 -> [w392 w403]
            tunnel: [w392 w403] -> w385
            tunnel: [w389 w400] -> w384
            tunnel: w383 -> [w390 w401]
            frame False {
              w394 = T7[] [5, 9] items=["DO 0 [KP1] [M12]", "DO 1 [ON KP2] [M21]", "DO 2 [ON KP3] [M24]", "DO 3 [WATER Y18.1 [DO3]]", "DO 4 [WATER Y18.2 [DO4]]", "DO 5 [KP6 Y29.1 33.7]", "DO 6 [KP7 Y29.2 33.8]", "DO 7 [KP8 Y29.3 33.9]", "DO 8 [KP9 Y29.4  33.12]", "DO 9 [KP10 Y29.5 33.1]", "DO 10 [KP11 Y29.6 33.2]", "DO 11 [KP12 Y29.7  33.13]", "DO 12 [KP13 Y29.8  33.11]", "DO 13 [KP14 Y29.9 33.10]", "DO 14 [KP15 Y29.10  33.6]", "DO 15 [KP16 Y29.11  33.5]", "DO 16 [KP17 Y29.12  33.4]", "DO 17 [KP18 Y29.13 33.3]", "DO 18 [AIR KP19]", "DO 19 [STEP DRIVE EN KP20]", "DO 20 [KP21 Y44.1 OPEN]", "DO 21 [ KP22 Y44.1 CLOSE]", "DO 22 [ KP23 Y44.2 OPEN]", "DO 23", "DO 24 [STEP DRIVE 1]", "DO 25 [STEP DRIVE 2]"] ("#DO")
              (unwired) TRUE ("Do")
              n154 = call "GetFPGA.vi"("Device in"=w392) -> ("FPGA API.lvclass"=w398:refnum<class "FPGA API.lvclass">)  [unwired: 10 in]
              n155 = call-dynamic "SetHasckelAO.vi"("FPGA API in"=w398, "Haskel in"=0.0, "error in (no error)"=w390) -> ("FPGA API out"=w396:refnum<class "FPGA API.lvclass">, "error out"=w397:errorcluster)  [unwired: 11 in]
              n156 = call "DoValve.vi"("#DO"=w394, "error in (no error)"=w397, "reference in"=w396) -> ("error out"=w399:errorcluster, "reference out"=w391:refnum<class "FPGA API.lvclass">)  [unwired: 7 in]
              n157 = call-dynamic "SetPropValve.vi"("FPGA API in"=w391, "error in (no error)"=w399, "AO 1"=5.0) -> ("error out"=w389:errorcluster)  [unwired: 11 in, 1 out]
            }
            frame True {
              w404 = T7[] [9] items=["DO 0 [KP1] [M12]", "DO 1 [ON KP2] [M21]", "DO 2 [ON KP3] [M24]", "DO 3 [WATER Y18.1 [DO3]]", "DO 4 [WATER Y18.2 [DO4]]", "DO 5 [KP6 Y29.1 33.7]", "DO 6 [KP7 Y29.2 33.8]", "DO 7 [KP8 Y29.3 33.9]", "DO 8 [KP9 Y29.4  33.12]", "DO 9 [KP10 Y29.5 33.1]", "DO 10 [KP11 Y29.6 33.2]", "DO 11 [KP12 Y29.7  33.13]", "DO 12 [KP13 Y29.8  33.11]", "DO 13 [KP14 Y29.9 33.10]", "DO 14 [KP15 Y29.10  33.6]", "DO 15 [KP16 Y29.11  33.5]", "DO 16 [KP17 Y29.12  33.4]", "DO 17 [KP18 Y29.13 33.3]", "DO 18 [AIR KP19]", "DO 19 [STEP DRIVE EN KP20]", "DO 20 [KP21 Y44.1 OPEN]", "DO 21 [ KP22 Y44.1 CLOSE]", "DO 22 [ KP23 Y44.2 OPEN]", "DO 23", "DO 24 [STEP DRIVE 1]", "DO 25 [STEP DRIVE 2]"] ("#DO")
              (unwired) TRUE ("Do")
              n158 = call "GetFPGA.vi"("Device in"=w403) -> ("FPGA API.lvclass"=w406:refnum<class "FPGA API.lvclass">)  [unwired: 10 in]
              n159 = call "DoValve.vi"("#DO"=w404, "error in (no error)"=w401, "reference in"=w406) -> ("error out"=w407:errorcluster, "reference out"=w402:refnum<class "FPGA API.lvclass">)  [unwired: 7 in]
              n160 = call-dynamic "SetPropValve.vi"("FPGA API in"=w402, "error in (no error)"=w407, "AO 1"=0.0) -> ("error out"=w400:errorcluster)  [unwired: 11 in, 1 out]
            }
          }
        }
        frame "Pressure pre loading: Chamber" {
          n161 = call "Get PV.vi"("Stand in"=w412) -> ("Stat Data.scl mean"=w414:dbl)  [unwired: 10 in]
          n162 = Greater?(x=w414, y=3.0) -> (0:w408:bool)
          n163 = case shown="True" w408 {
            tunnel: w412 -> [w418 w429]
            tunnel: [w418 w429] -> w411
            tunnel: [w415 w426] -> w410
            tunnel: w409 -> [w416 w427]
            frame False {
              w420 = T7[] [5, 10] items=["DO 0 [KP1] [M12]", "DO 1 [ON KP2] [M21]", "DO 2 [ON KP3] [M24]", "DO 3 [WATER Y18.1 [DO3]]", "DO 4 [WATER Y18.2 [DO4]]", "DO 5 [KP6 Y29.1 33.7]", "DO 6 [KP7 Y29.2 33.8]", "DO 7 [KP8 Y29.3 33.9]", "DO 8 [KP9 Y29.4  33.12]", "DO 9 [KP10 Y29.5 33.1]", "DO 10 [KP11 Y29.6 33.2]", "DO 11 [KP12 Y29.7  33.13]", "DO 12 [KP13 Y29.8  33.11]", "DO 13 [KP14 Y29.9 33.10]", "DO 14 [KP15 Y29.10  33.6]", "DO 15 [KP16 Y29.11  33.5]", "DO 16 [KP17 Y29.12  33.4]", "DO 17 [KP18 Y29.13 33.3]", "DO 18 [AIR KP19]", "DO 19 [STEP DRIVE EN KP20]", "DO 20 [KP21 Y44.1 OPEN]", "DO 21 [ KP22 Y44.1 CLOSE]", "DO 22 [ KP23 Y44.2 OPEN]", "DO 23", "DO 24 [STEP DRIVE 1]", "DO 25 [STEP DRIVE 2]"] ("#DO")
              (unwired) TRUE ("Do")
              n164 = call "GetFPGA.vi"("Device in"=w418) -> ("FPGA API.lvclass"=w424:refnum<class "FPGA API.lvclass">)  [unwired: 10 in]
              n165 = call-dynamic "SetHasckelAO.vi"("FPGA API in"=w424, "Haskel in"=0.0, "error in (no error)"=w416) -> ("FPGA API out"=w422:refnum<class "FPGA API.lvclass">, "error out"=w423:errorcluster)  [unwired: 11 in]
              n166 = call "DoValve.vi"("#DO"=w420, "error in (no error)"=w423, "reference in"=w422) -> ("error out"=w425:errorcluster, "reference out"=w417:refnum<class "FPGA API.lvclass">)  [unwired: 7 in]
              n167 = call-dynamic "SetPropValve.vi"("FPGA API in"=w417, "error in (no error)"=w425, "AO 1"=5.0) -> ("error out"=w415:errorcluster)  [unwired: 11 in, 1 out]
            }
            frame True {
              w430 = T7[] [10] items=["DO 0 [KP1] [M12]", "DO 1 [ON KP2] [M21]", "DO 2 [ON KP3] [M24]", "DO 3 [WATER Y18.1 [DO3]]", "DO 4 [WATER Y18.2 [DO4]]", "DO 5 [KP6 Y29.1 33.7]", "DO 6 [KP7 Y29.2 33.8]", "DO 7 [KP8 Y29.3 33.9]", "DO 8 [KP9 Y29.4  33.12]", "DO 9 [KP10 Y29.5 33.1]", "DO 10 [KP11 Y29.6 33.2]", "DO 11 [KP12 Y29.7  33.13]", "DO 12 [KP13 Y29.8  33.11]", "DO 13 [KP14 Y29.9 33.10]", "DO 14 [KP15 Y29.10  33.6]", "DO 15 [KP16 Y29.11  33.5]", "DO 16 [KP17 Y29.12  33.4]", "DO 17 [KP18 Y29.13 33.3]", "DO 18 [AIR KP19]", "DO 19 [STEP DRIVE EN KP20]", "DO 20 [KP21 Y44.1 OPEN]", "DO 21 [ KP22 Y44.1 CLOSE]", "DO 22 [ KP23 Y44.2 OPEN]", "DO 23", "DO 24 [STEP DRIVE 1]", "DO 25 [STEP DRIVE 2]"] ("#DO")
              n168 = call "GetFPGA.vi"("Device in"=w429) -> ("FPGA API.lvclass"=w432:refnum<class "FPGA API.lvclass">)  [unwired: 10 in]
              n169 = call "DoValve.vi"("#DO"=w430, "error in (no error)"=w427, "reference in"=w432) -> ("error out"=w433:errorcluster, "reference out"=w428:refnum<class "FPGA API.lvclass">)  [unwired: 7 in]
              n170 = call-dynamic "SetPropValve.vi"("FPGA API in"=w428, "error in (no error)"=w433, "AO 1"=0.0) -> ("error out"=w426:errorcluster)  [unwired: 11 in, 1 out]
            }
          }
        }
        frame "Slow Pressure Release: In Progress (DUT)" {
          n171 = Unbundle By Name(w434) -> ("Pressure SP"=w444:dbl)
          n172 = Unbundle By Name(w434) -> ("NV_DUT"=w442:refnum<class "NeedleValve.lvclass">)
          n173 = call "Get PV.vi"("Stand in"=w434) -> ("Stat Data.scl mean"=w445:dbl)  [unwired: 10 in]
          n174 = call "Read Data.vi"("NeedleValve in"=w442) -> ("data value"=w439:T14)  [unwired: 10 in]
          n175 = Less Or Equal?(x=w445, y=w444) -> (x <= y?=w443:bool)
          n176 = Unbundle By Name(w439) -> ("Angele"=w440:dbl)
          n177 = call "GetFPGA.vi"("Device in"=w434) -> ("FPGA API.lvclass"=w437:refnum<class "FPGA API.lvclass">)  [unwired: 10 in]
          n178 = Greater?(x=w440, y=40.0) -> (0:w441:bool)
          n179 = case shown="True" w441 {
            tunnel: [w446 w450] -> w435
            tunnel: w436 -> [w446 w449]
            tunnel: w437 -> [_ w448]
            frame False {
            }
            frame True {
              n180 = call-dynamic "Enable Stop Step.vi"("FPGA API in"=w448, "error in (no error)"=w449, "Direction"=Direction."DUT") -> ("error out"=w450:errorcluster)  [unwired: 11 in, 1 out]
            }
          }
        }
        frame "Slow Pressure Release: In Progress (Chamber)" {
          n181 = Unbundle By Name(w451) -> ("NV_Chamber"=w459:refnum<class "NeedleValve.lvclass">)
          n182 = Unbundle By Name(w451) -> ("Pressure SP"=w461:dbl)
          n183 = call "Get PV.vi"("Stand in"=w451) -> ("Stat Data.scl mean"=w462:dbl)  [unwired: 10 in]
          n184 = call "Read Data.vi"("NeedleValve in"=w459) -> ("data value"=w456:T14)  [unwired: 10 in]
          n185 = Less Or Equal?(x=w462, y=w461) -> (x <= y?=w460:bool)
          n186 = Unbundle By Name(w456) -> ("Angele"=w457:dbl)
          n187 = call "GetFPGA.vi"("Device in"=w451) -> ("FPGA API.lvclass"=w454:refnum<class "FPGA API.lvclass">)  [unwired: 10 in]
          n188 = Greater?(x=w457, y=40.0) -> (0:w458:bool)
          n189 = case shown="True" w458 {
            tunnel: [w463 w467] -> w452
            tunnel: w453 -> [w463 w466]
            tunnel: w454 -> [_ w465]
            frame False {
            }
            frame True {
              n190 = call-dynamic "Enable Stop Step.vi"("FPGA API in"=w465, "error in (no error)"=w466, "Direction"=Direction."Chamber") -> ("error out"=w467:errorcluster)  [unwired: 11 in, 1 out]
            }
          }
        }
      }
      n191 = case shown="True" w12 {
        tunnel: [w468 w469] -> w11
        tunnel: w10 -> [w468 w470]
        frame False {
        }
        frame True {
          n192 = in-place {
            n193 = in-place-cluster #12(w470) -> ("Actions"=w473:T1[])
            n194 = Delete From Array(array=w473, index=0) -> (array with subset deleted=w472:T1[])  [unwired: 1 in, 1 out]
            n195 = in-place-cluster #12("Actions"=w472) -> (w469:refnum<class "Stand.lvclass">)
          }
        }
      }
    }
    frame True {
      n196 = Bundle By Name(cluster=w477, "Action"=Action."NONE" ("Data.Action")) -> (w475:refnum<class "Stand.lvclass">)
    }
  }
  "error out" <- w5
  "Stand out" <- w6
